vi "Update_Dust_Info.vi"() -> ()   [LabVIEW 2013]
doc: "Updates the dust_info and dust_info_small tables. For use in the Dust Lab, so anyone changing the source can update the database with the new source before going downstairs."
uses:
  <userlib>/Accelerator/User Interface/Controls/Dust_Properties.ctl
  <userlib>/Accelerator/User Interface/Controls/source_builders.ctl
  <userlib>/Accelerator/User Interface/Controls/dust_type_indicator.ctl
  <vilib>/Utility/miscctls.llb/LVPointTypeDef.ctl
panel:
  in  "error in (no error)":errorcluster
  out "error out":errorcluster
  in  "Exit":bool
  in  "Clear Errors":bool
  out "Dust Properties small":T1
  in  "Update dust info small":bool
  out "Dust Type small":T2 {"Batch" step=1; "Type" step=1; "Dust Source Builder:" items=["Keith Drake", "Nick Beaty", "Anthony Shu", "David James", "John Fontanese"]}
  out "Dust Properties":T1
  in  "Update dust info":bool
  out "Dust Type":T2 {"Batch" step=1; "Type" step=1; "Dust Source Builder:" items=["Keith Drake", "Nick Beaty", "Anthony Shu", "David James", "John Fontanese"]}
  # "Dust Information - Small"
  # "Dust Information - Big"
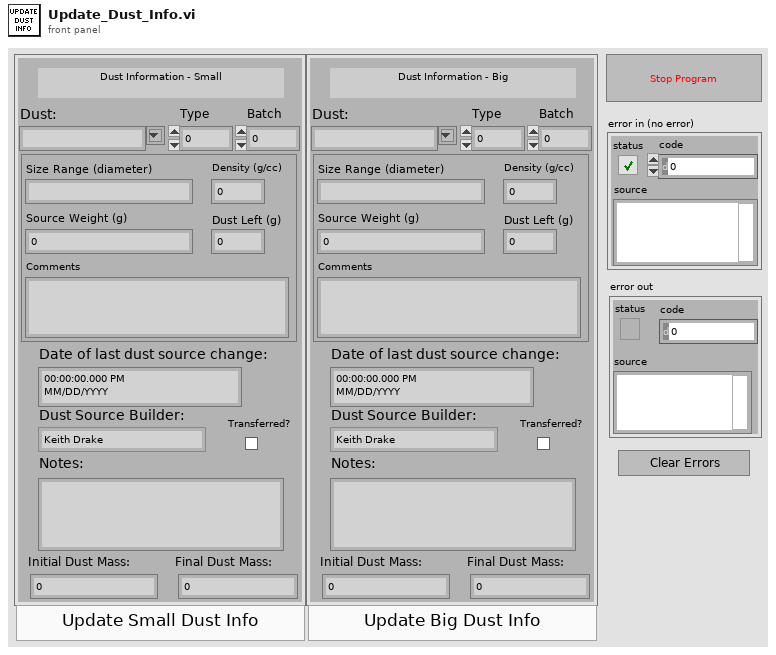
[diagram p1: front panel]
types:
  T1 = typedef "dust_type_indicator.ctl" = cluster{"id_dust_type":i32, "Size Range (diameter)":string, "Density (g/cc)":dbl, "Source Weight (g)":dbl, "Dust Left (g)":dbl, "Comments":string}
  T2 = typedef "Dust_Properties.ctl" = cluster{"Dust info id":u16, "Integer Timestamp":i64, "Dust:":string, "Dust Source Builder:":T3, "Notes:":string, "Date of last dust source change:":timestamp, "Initial Dust Mass:":dbl, "Final Dust Mass:":dbl, "Type":u16, "Batch":u16, "dust type id":u16, "Transferred?":bool}
  T3 = typedef "source_builders.ctl" = u16
  T4 = typedef "LVPointTypeDef.ctl" = cluster{"Horizontal":i16, "Vertical":i16}
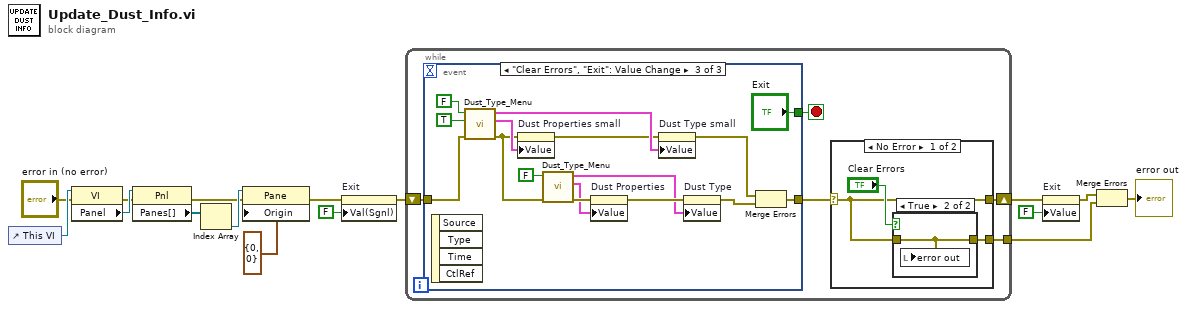
[diagram p0: block diagram]
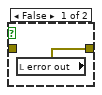
[diagram p2: hidden frame]
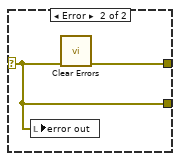
[diagram p3: hidden frame]
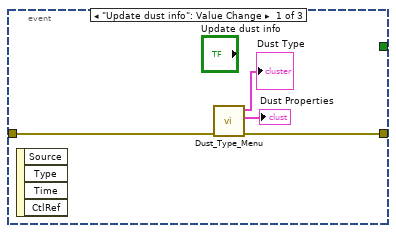
[diagram p4: hidden frame]
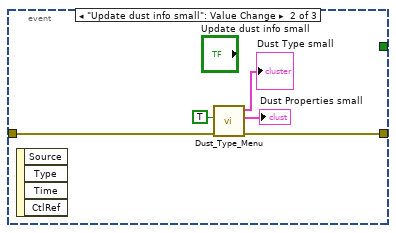
[diagram p5: hidden frame]
diagram:
  n1 = control-ref of="This VI"() -> (w9:refnum<vi>)
  n2 = property class="VI"(reference=w9, error in="error in (no error)") -> (error out=w10:errorcluster, "Panel"=w11:refnum<vi>)  [unwired: 1 out]
  n3 = property class="Pnl"(reference=w11, error in=w10) -> (error out=w12:errorcluster, "Panes[]"=w13:refnum<vi>[])  [unwired: 1 out]
  n4 = Index Array(array=w13) -> (element=w14:refnum<vi>)  [unwired: 1 in]
  n5 = property class="Pane"(reference=w14, error in=w12, "Origin"=T4 {"Horizontal"=0, "Vertical"=0}) -> (error out=w1:errorcluster)  [unwired: 1 out]
  n6 = property on="Exit" class="Bool (strict)"(error in=w1, "Val(Sgnl)"=FALSE ("Exit")) -> (error out=w6:errorcluster)  [unwired: 1 in, 1 out]
  n7 = while {
    shift-right: [w19] -> w4
    shift-left: w6 -> [w17]
    tunnel: [w18] -> w16
    stop <- w21 stop-if-true
    n8 = event shown="[2] \"Clear Errors\", \"Exit\": Value Change" {
      selector: _ -> [_ _ _]
      dyn-events: _ -> [_ _ _]
      timeout: _ -> [_ _ _]
      tunnel: w17 -> [w31 w36 w42]
      tunnel: [w32 w37 w39] -> w20
      tunnel: [_ _ "Exit"] -> w21
      event "Update dust info": Value Change {
        n9 = event-data() -> ()  [unwired: 1 in, 4 out]
        n10 = call <userlib>:"Dust_Type_Menu.vi"("error in (no error)"=w31) -> ("error out"=w32:errorcluster, "Dust Properties"=→"Dust Properties":T1, "Dust Info"=→"Dust Type":T2)  [unwired: 7 in, 1 out]
      }
      event "Update dust info small": Value Change {
        n11 = event-data() -> ()  [unwired: 1 in, 4 out]
        n12 = call <userlib>:"Dust_Type_Menu.vi"("error in (no error)"=w36, "Small?"=TRUE ("Sub vi?")) -> ("error out"=w37:errorcluster, "Dust Properties"=→"Dust Properties small":T1, "Dust Info"=→"Dust Type small":T2)  [unwired: 6 in, 1 out]
      }
      event "Clear Errors", "Exit": Value Change {
        n13 = event-data() -> ()  [unwired: 1 in, 4 out]
        n14 = call <userlib>:"Dust_Type_Menu.vi"("error in (no error)"=w42, "Small?"=TRUE, "Enable"=FALSE) -> ("error out"=w38:errorcluster, "Dust Properties"=w51:T1, "Dust Info"=w52:T2)  [unwired: 5 in, 1 out]
        n15 = property on="Dust Properties small" class="Clust (strict)"(error in=w38, "Value"=w51) -> (error out=w43:errorcluster)  [unwired: 1 in, 1 out]
        n16 = call <userlib>:"Dust_Type_Menu.vi"("error in (no error)"=w38, "Enable"=FALSE) -> ("error out"=w48:errorcluster, "Dust Properties"=w46:T1, "Dust Info"=w45:T2)  [unwired: 6 in, 1 out]
        n17 = property on="Dust Properties" class="Clust (strict)"(error in=w48, "Value"=w46) -> (error out=w47:errorcluster)  [unwired: 1 in, 1 out]
        n18 = property on="Dust Type small" class="Clust (strict)"(error in=w43, "Value"=w52) -> (error out=w41:errorcluster)  [unwired: 1 in, 1 out]
        n19 = property on="Dust Type" class="Clust (strict)"(error in=w47, "Value"=w45) -> (error out=w40:errorcluster)  [unwired: 1 in, 1 out]
        n20 = Merge Errors(w41, w40) -> (w39:errorcluster)
      }
    }
    n21 = case shown="No Error" w20 {
      selector: w20 -> [w23 w27]
      tunnel: [w23 w28] -> w19
      tunnel: [w22 w27] -> w18
      frame No Error {
        n22 = case shown="True" "Clear Errors" {
          tunnel: w23 -> [_ w26]
          tunnel: [w25 w26] -> w22
          frame False {
            n23 = local read "error out"() -> (w25:errorcluster)
          }
          frame True {
            n24 = local write "error out"(w26) -> ()
          }
        }
      }
      frame Error {
        n25 = local write "error out"(w27) -> ()
        n26 = call <vilib>:"Clear Errors.vi"("error in (no error)"=w27) -> ("error out"=w28:errorcluster)  [unwired: 6 in]
      }
    }
  }
  n27 = property on="Exit" class="Bool (strict)"(error in=w4, "Value"=FALSE ("Exit")) -> (error out=w2:errorcluster)  [unwired: 1 in, 1 out]
  n28 = Merge Errors(w2, w16) -> (→"error out":errorcluster)
